vi "File.Create UUT Dir.vi"(7 "Start Time":timestamp, 10 "SN":string="ABC123", 11 "Local Data Dir":path) -> (2 "error out":errorcluster, 3 "UUTDir":path, 5 "SN_Time":string)   [LabVIEW 2018]
uses:
  Errors/Error.Error Code List.ctl
  <vilib>/KATE/Files/File Utils.lvlib
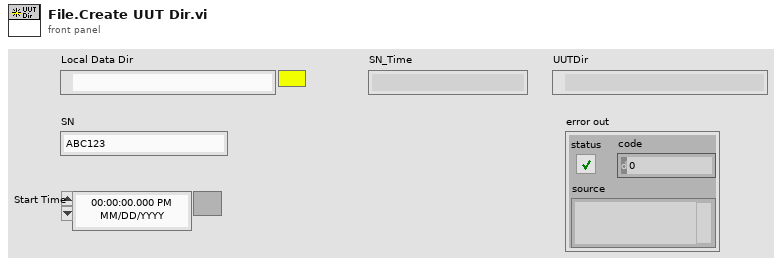
[diagram p1: front panel]
types:
  T1 = typedef "Error.Error Code List.ctl" = i32
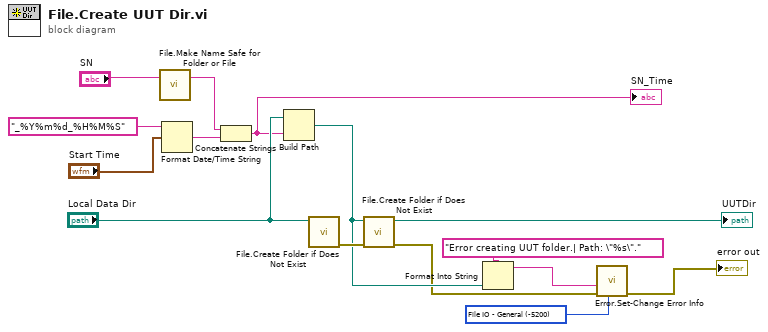
[diagram p0: block diagram]
diagram:
  w7 = T1 -5200 items=["No Error"=0, "Abort"=-2, "Misc"=-5000, "Fixture Error"=-5100, "File IO - General"=-5200, "FIle IO - Config Error"=-5201, "Instrument - General"=-5300, "Instrument - Serial Com"=-5301, "Instrument - Camera"=-5302, "Instrument - PS"=-5303, "Instrument - Oscilloscope"=-5304, "Instrument - Function Gen"=-5305, "Instrument - Load"=-5306, "Instrument - Meter"=-5307, "Instrument - Power Control"=-5308, "Instrument - Motion"=-5309, "Instrument - RF"=-5310, "System Exe"=-5400, "Image Processing"=-5500, "Communication"=-5600, "Script - Syntax Error"=-6000, "Script - Invalid Name or Param"=-6100, "Script - Timeout"=-6200, "Invalid Data"=-6300] ("Std Code")
  n1 = call <vilib>:"File.Make Name Safe for Folder or File.vi"("File Name"="SN") -> ("Fixed Name"=w1:string)  [unwired: 2 in]
  n2 = Format Date/Time String(time format string (%c)="_%Y%m%d_%H%M%S", seconds (now)="Start Time") -> (date/time string=w10:string)  [unwired: 1 in]
  n3 = Concatenate Strings(w1, w10) -> (w3:string)
  "SN_Time" <- w3
  n4 = Build Path(base path="Local Data Dir", name or relative path=w3) -> (appended path=w6:path)
  n5 = call <vilib>:"File.Create Folder if Does Not Exist.vi"("Path"="Local Data Dir") -> ("error out"=w12:errorcluster)  [unwired: 8 in, 2 out]
  n6 = call <vilib>:"File.Create Folder if Does Not Exist.vi"("error in"=w12, "Path"=w6) -> ("error out"=w5:errorcluster, "Dup Path"=→"UUTDir":path)  [unwired: 7 in, 1 out]
  n7 = Format Into String(format string="Error creating UUT folder.| Path: \"%s\".", w6) -> (resulting string=w8:string)  [unwired: 2 in, 1 out]
  n8 = call "Error.Set-Change Error Info.vi"("Std Code"=w7, "error in"=w5, "Description"=w8) -> ("error out"=→"error out":errorcluster)  [unwired: 8 in]
